vi "1L12-tb-conv-tab1D-en-tab2D.vi"(1 "tab 1D":dbl[](array[numeric]), 2 "Taille ligne":i32=5) -> (0 "tab 2D":dbl[][](array[numeric]))   [LabVIEW 2010, in "lv_01.lvlib"]
uses:
  lv_01.lvlib
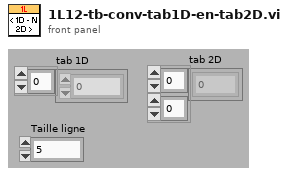
[diagram p1: front panel]
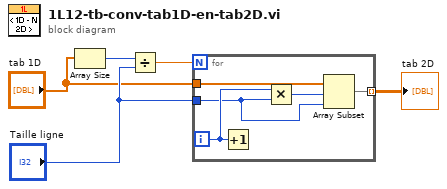
[diagram p0: block diagram]
diagram:
  n1 = Array Size(array="tab 1D") -> (size(s)=w3:i32)
  n2 = Divide(x=w3, y="Taille ligne") -> (x/y=w5:dbl)
  n3 = for {
    N: w5 -> [_]
    tunnel: "tab 1D" -> [w8]
    tunnel: [w7] -> w1 mode=indexing
    tunnel: "Taille ligne" -> [w6]
    i -> [w10]
    n4 = Increment(x=w10) -> ()  [unwired: 1 out]
    n5 = Multiply(x=w10, y=w6) -> (x*y=w9:i32)
    n6 = Array Subset(array=w8, index=w9, length=w6) -> (w7:dbl[])
  }
  "tab 2D" <- w1
